vi "bitmanip.vi"(0 "Pulse Type":u16(ring) items=["Header Information", "Particle Pulse", "Test Pulse"], 1 "Integer to be written":i16 format="%16.0f") -> (3 "Integer Written":i16)   [LabVIEW 2012]
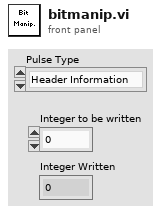
[diagram p1: front panel]
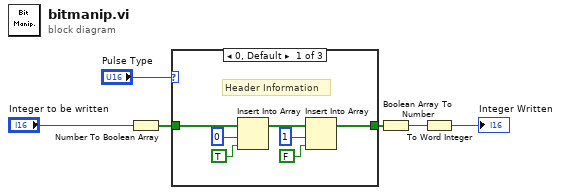
[diagram p0: block diagram]
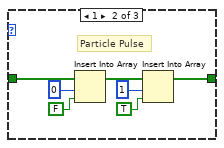
[diagram p2: hidden frame]
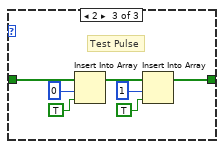
[diagram p3: hidden frame]
diagram:
  n1 = Number To Boolean Array(number="Integer to be written") -> (Boolean array=w4:bool[])
  n2 = case shown="0, Default" "Pulse Type" {
    tunnel: w4 -> [w8 w15 w22]
    tunnel: [w7 w14 w21] -> w3
    frame 0, Default {
      # "Header Information"
      n3 = Insert Into Array(array=w8, index=0, new element=TRUE ("new element/subarray")) -> (w11:bool[])
      n4 = Insert Into Array(array=w11, index=1, new element=FALSE ("new element/subarray")) -> (w7:bool[])
    }
    frame 1 {
      # "Particle Pulse"
      n5 = Insert Into Array(array=w15, index=0, new element=FALSE ("new element/subarray")) -> (w18:bool[])
      n6 = Insert Into Array(array=w18, index=1, new element=TRUE ("new element/subarray")) -> (w14:bool[])
    }
    frame 2 {
      # "Test Pulse"
      n7 = Insert Into Array(array=w22, index=0, new element=TRUE ("new element/subarray")) -> (w25:bool[])
      n8 = Insert Into Array(array=w25, index=1, new element=TRUE ("new element/subarray")) -> (w21:bool[])
    }
  }
  n9 = Boolean Array To Number(Boolean array=w3) -> (number=w2:u32)
  n10 = To Word Integer(number=w2) -> (16bit integer=→"Integer Written":i16)
